vi "getTimeChannelFromXmlNative.vi"(8 "error in (no error)":errorcluster, 10 "eventXML":refnum<k20>, 11 "ScriptEvent in":refnum<class "ScriptEvent.lvclass">) -> (0 "error out":errorcluster, 2 "eventXML out":refnum<k20>, 3 "ScriptEvent out":refnum<class "ScriptEvent.lvclass">)   [LabVIEW 2009, in "Tools.lvlib" / "Scripting.lvlib" / "ScriptEvent.lvclass"]
uses:
  ScriptEvent.lvclass
  DatabaseHelpers/Database Objects/Channel/Channel.lvclass
  <vilib>/xml/Close Reference(NNMap).vi
  <vilib>/xml/Close Reference(Node).vi
  Program Files/National Instruments/LabVIEW 2009/resource/objmgr/DOMUserDefRef.rc
  <vilib>/xml/NI_XML.lvlib
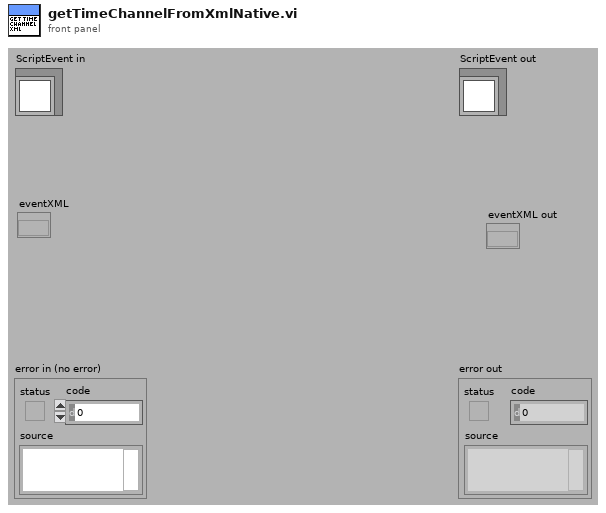
[diagram p1: front panel]
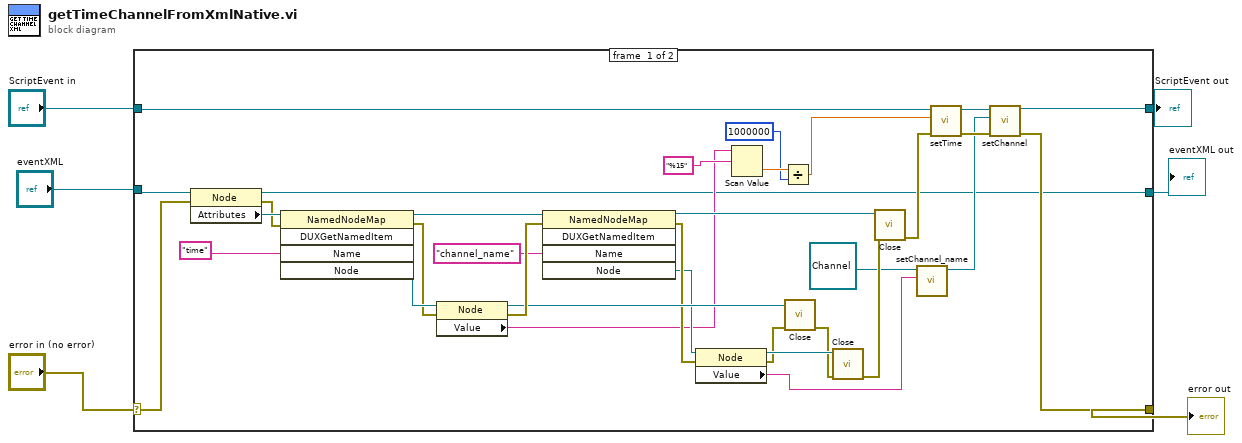
[diagram p0: block diagram]
diagram:
  n1 = case shown="No Error" "error in (no error)" {
    selector: "error in (no error)" -> [w13 w41]
    tunnel: [w14 w41] -> w5
    tunnel: [w15 w40] -> w3
    tunnel: "ScriptEvent in" -> [w16 w40]
    tunnel: "eventXML" -> [w39 _]
    tunnel: [w7 _] -> w1
    frame #0 {
      n2 = property class="Node"(reference=w39, error in=w13) -> (reference out=w7:refnum<k20>, error out=w35:errorcluster, "Attributes"=w36:refnum<k20>)
      n3 = invoke class="NamedNodeMap" method="DUXGetNamedItem"(reference=w36, error in=w35, "Name"="time") -> (reference out=w34:refnum<k20>, error out=w37:errorcluster, "Node"=w38:refnum<k20>)  [unwired: 2 in, 2 out]
      n4 = property class="Node"(reference=w38, error in=w37) -> (reference out=w32:refnum<k20>, error out=w33:errorcluster, "Value"=w21:string)
      n5 = invoke class="NamedNodeMap" method="DUXGetNamedItem"(reference=w34, error in=w33, "Name"="channel_name") -> (reference out=w27:refnum<k20>, error out=w26:errorcluster, "Node"=w25:refnum<k20>)  [unwired: 2 in, 2 out]
      n6 = property class="Node"(reference=w25, error in=w26) -> (reference out=w31:refnum<k20>, error out=w30:errorcluster, "Value"=w9:string)
      n7 = Scan Value(string=w21, format string="%15") -> (value=w20:dbl)  [unwired: 1 in, 1 out]
      n8 = Divide(x=w20, y=1000000) -> (x/y=w12:dbl)
      n9 = call-poly <vilib>:"Close.vi"("error in (no error)"=w30, "node"=w32) -> ("error out"=w29:errorcluster)  [unwired: 7 in]
      n10 = call-poly <vilib>:"Close.vi"("error in (no error)"=w29, "node"=w31) -> ("error out"=w28:errorcluster)  [unwired: 7 in]
      n11 = call-poly <vilib>:"Close.vi"("error in (no error)"=w28, "named node map"=w27) -> ("error out"=w11:errorcluster)  [unwired: 7 in]
      n12 = call "setChannel_name.vi"("channel_name"=w9, "Channel.lvclass in"=refnum<class "Channel.lvclass"> refnum ("Tools.lvlib:DatabaseHelpers.lvlib:Channel.lvclass")) -> ("Channel.lvclass out"=w8:refnum<class "Channel.lvclass">)  [unwired: 8 in, 1 out]
      n13 = call "setTime.vi"("error in (no error)"=w11, "time"=w12, "ScriptEvent.lvclass in"=w16) -> ("error out"=w17:errorcluster, "ScriptEvent.lvclass out"=w18:refnum<class "ScriptEvent.lvclass">)  [unwired: 7 in]
      n14 = call-dynamic "setChannel.vi"("error in (no error)"=w17, "Channel.lvclass"=w8, "ScriptEvent.lvclass in"=w18) -> ("error out"=w14:errorcluster, "ScriptEvent.lvclass out"=w15:refnum<class "ScriptEvent.lvclass">)  [unwired: 7 in]
    }
    frame #1 {
    }
  }
  "error out" <- w5
  "ScriptEvent out" <- w3
  "eventXML out" <- w1
